vi "simulate ext start.vi"(8 "error in (no error)":errorcluster, 10 "encoder":i16, 11 "delay":i16) -> (0 "error out":errorcluster)   [LabVIEW 2015, in "SCANalone4x64.lvlib"]
doc: "__declspec(dllimport) void __stdcall simulate_ext_start(short delay, short encoder);"
uses:
  <userlib>/SCANalone4x64/SCANalone4x64.lvlib
  <userlib>/SCANalone4x64/SCANalone4x64.dll
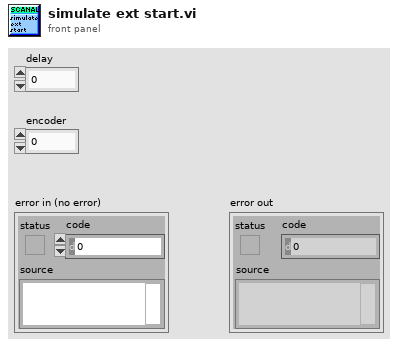
[diagram p1: front panel]
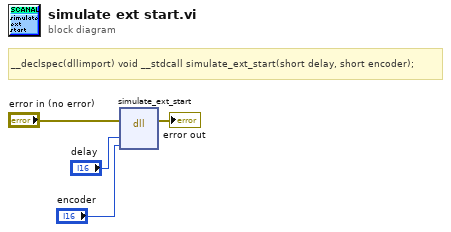
[diagram p0: block diagram]
diagram:
  # "__declspec(dllimport) void __stdcall simulate_ext_start(short delay, short encoder);"
  n1 = dll-call lib="C:/Program Files/National Instruments/LabVIEW 2015/user.lib/SCANalone4x64/SCANalone4x64.*" fn="simulate_ext_start"(error in="error in (no error)", "delay"="delay", "encoder"="encoder") -> (error out=→"error out":errorcluster)  [unwired: 5 in, 1 out]
